vi "Sync Out (TDM).vi"(5 "sync mode":T1, 6 "channel count (2)":u8=2, 7 "bit set edge (falling)":enum16{"rising", "falling"}(ring)=enum."falling", 9 "ready for input?":bool, 10 "transmit":bool, 11 "clock in":bool) -> (1 "ready for input":bool, 2 "latch config":bool, 3 "frame sync":bool)   [LabVIEW 2013, in "I2S-TDM.lvlib"]
uses:
  I2S-TDM.lvlib
  Controls/sync modes.ctl
  Controls/frame sync states.ctl
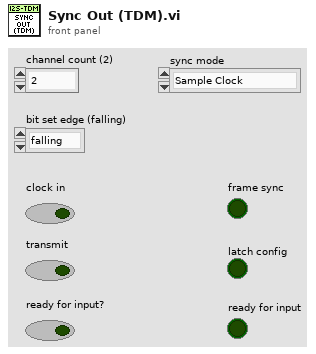
[diagram p1: front panel]
types:
  T1 = typedef "I2S-TDM.lvlib/sync modes.ctl" = enum16{"Sample Clock", "Pulse"}
  T2 = typedef "I2S-TDM.lvlib/frame sync states.ctl" = enum16{"idle", "pre-transfer", "transfer"}
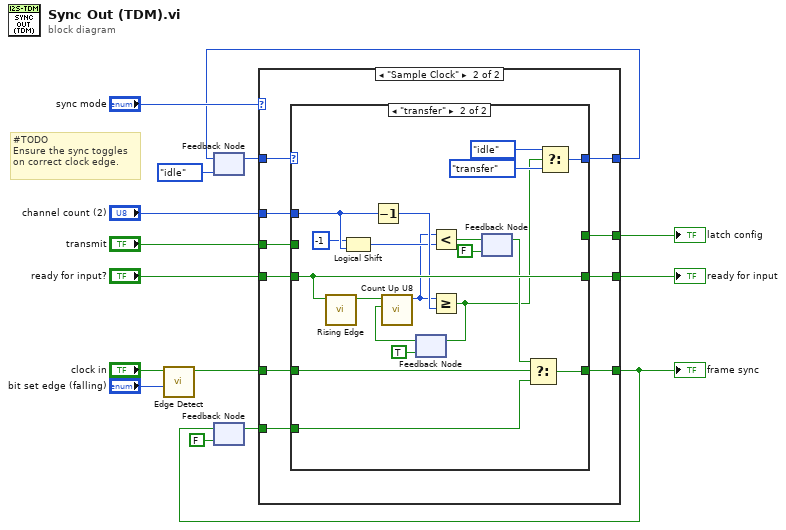
[diagram p0: block diagram]
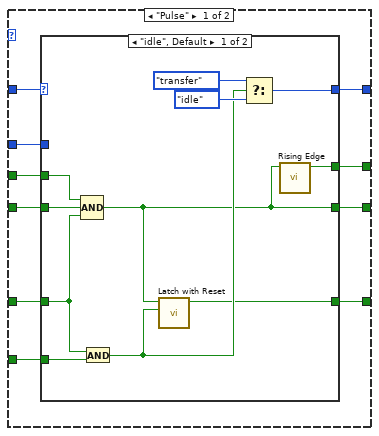
[diagram p2: hidden frame]
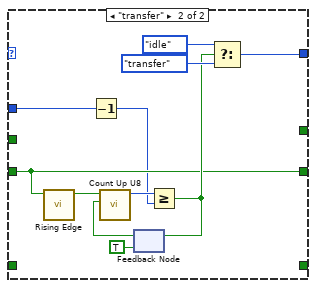
[diagram p3: hidden frame]
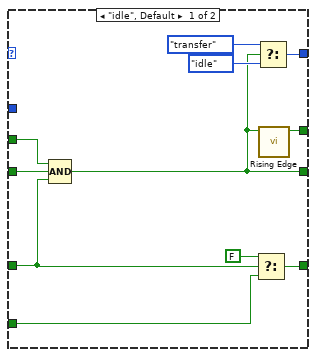
[diagram p4: hidden frame]
diagram:
  # "#TODO\nEnsure the sync toggles on correct clock edge."
  n1 = call "Edge Detect.vi"("edge (rising)"="bit set edge (falling)", "signal in"="clock in") -> ("edge detected?"=w10:bool)  [unwired: 9 in]
  n2 = feedback #1(frame_sync_states."idle") -> (w14:T2)
  n3 = feedback #2(FALSE ("latched signal")) -> (w6:bool)
  n4 = case shown="\"Sample Clock\"" "sync mode" {
    tunnel: w14 -> [w25 w57]
    tunnel: "ready for input?" -> [w24 w56]
    tunnel: w10 -> [w23 w55]
    tunnel: [w22 w54] -> w9
    tunnel: "transmit" -> [w21 w53]
    tunnel: [w20 w52] -> w7
    tunnel: [w19 w51] -> w2
    tunnel: w6 -> [w18 w50]
    tunnel: "channel count (2)" -> [w17 w49]
    tunnel: [w16 w48] -> w3
    frame "Pulse" {
      n5 = case shown="\"idle\", Default" w25 {
        tunnel: [w34 w45] -> w16
        tunnel: w21 -> [w32 _]
        tunnel: w24 -> [w31 w39]
        tunnel: w23 -> [w29 _]
        tunnel: [w26 w39] -> w22
        tunnel: [w27 _] -> w19
        tunnel: w17 -> [_ w38]
        tunnel: [w30 _] -> w20
        tunnel: w18 -> [w33 _]
        frame "idle", Default {
          n6 = Compound Arithmetic op=AND(w32, w31, w29) -> (w26:bool)
          n7 = And(x=w29, y=w33) -> (x .and. y?=w28:bool)
          n8 = call "Latch with Reset.vi"("reset"=w28, "signal"=w26) -> ("latched signal"=w27:bool)  [unwired: 9 in]
          n9 = Select(t=frame_sync_states."transfer", s=w28, f=frame_sync_states."idle") -> (s? t:f=w34:T2)
          n10 = call "Rising Edge.vi"("signal in"=w26) -> ("rising edge?"=w30:bool)  [unwired: 10 in]
        }
        frame "transfer" {
          n11 = call "Rising Edge.vi"("signal in"=w39) -> ("rising edge?"=w44:bool)  [unwired: 10 in]
          n12 = Decrement(x=w38) -> (x-1=w37:u8)
          n13 = feedback #3(TRUE ("latched signal")) -> (w41:bool)
          n14 = call "Count Up U8.vi"("reset (F)"=w41, "increment"=w44) -> ("count"=w43:u8)  [unwired: 9 in]
          n15 = Greater Or Equal?(x=w43, y=w37) -> (x >= y?=w40:bool)
          n16 = feedback-in #3(w40) -> ()
          n17 = Select(t=frame_sync_states."idle", s=w40, f=frame_sync_states."transfer") -> (s? t:f=w45:T2)
        }
      }
    }
    frame "Sample Clock" {
      n18 = case shown="\"transfer\"" w57 {
        tunnel: [w66 w85] -> w48
        tunnel: w53 -> [w65 _]
        tunnel: w56 -> [w64 w81]
        tunnel: w55 -> [w59 w71]
        tunnel: [w62 w81] -> w54
        tunnel: [w60 w72] -> w51
        tunnel: w49 -> [_ w79]
        tunnel: [w63 _] -> w52
        tunnel: w50 -> [w58 w69]
        frame "idle", Default {
          n19 = Compound Arithmetic op=AND(w65, w64, w59) -> (w62:bool)
          n20 = Select(t=FALSE ("latched signal"), s=w59, f=w58) -> (s? t:f=w60:bool)
          n21 = Select(t=frame_sync_states."transfer", s=w62, f=frame_sync_states."idle") -> (s? t:f=w66:T2)
          n22 = call "Rising Edge.vi"("signal in"=w62) -> ("rising edge?"=w63:bool)  [unwired: 10 in]
        }
        frame "transfer" {
          n23 = call "Rising Edge.vi"("signal in"=w81) -> ("rising edge?"=w84:bool)  [unwired: 10 in]
          n24 = Logical Shift(y=i16 -1, x=w79) -> (x << y=w77:u8)
          n25 = Decrement(x=w79) -> (x-1=w80:u8)
          n26 = feedback #4(TRUE ("latched signal")) -> (w82:bool)
          n27 = call "Count Up U8.vi"("reset (F)"=w82, "increment"=w84) -> ("count"=w76:u8)  [unwired: 9 in]
          n28 = Less?(x=w76, y=w77) -> (x < y?=w75:bool)
          n29 = Greater Or Equal?(x=w76, y=w80) -> (x >= y?=w70:bool)
          n30 = feedback-in #4(w70) -> ()
          n31 = feedback-in #5(w75) -> ()
          n32 = feedback #5(FALSE) -> (w73:bool)
          n33 = Select(t=w73, s=w71, f=w69) -> (s? t:f=w72:bool)
          n34 = Select(t=frame_sync_states."idle", s=w70, f=frame_sync_states."transfer") -> (s? t:f=w85:T2)
        }
      }
    }
  }
  "ready for input" <- w9
  "frame sync" <- w2
  "latch config" <- w7
  n35 = feedback-in #1(w3) -> ()
  n36 = feedback-in #2(w2) -> ()
